vi "AlliGator Update Phasor Plot Image v2.vi"(5 "Image Control Refnum":T1 caption="Phasor Plot Display Refnum", 7 "Phasor Plot Color Scale":refnum<vi>, 8 "Error In":errorcluster, 9 "Phasor Plot Image Elements to Update":string[](array[string]), 10 "AlliGator Internal Variables DVR":refnum<data-value>, 11 "Phasor Plot Display Range Refnum":refnum<vi>) -> (0 "Error Out":errorcluster, 1 "Message":string, 2 "AlliGator Internal Variables DVR":refnum<data-value>)   [LabVIEW 2021, in "AlliGator Phasor Plot.lvlib"]
doc: "Updates the Phasor Plot image including its overlays."
uses:
  AlliGator Phasor Plot.lvlib
  AlliGator Internal Variables v2.ctl
  <vilib>/vision/Image Controls.llb/IMAQ Image.ctl
  AlliGator Gate Image Set.ctl
  AlliGator FLI Dataset Type.ctl
  AlliGator Data Series Type.ctl
  AlliGator Dataset Channel.ctl
  AlliGator Gate Arithmetic.ctl
  AlliGator Displayed Image.ctl
  Image/Named ROI Description.ctl
  AlliGator Decay Metadata v3.ctl
  AlliGator Decay Background Subtraction Info.ctl
  AlliGator Baseline Subtraction Method.ctl
  Graphs/XY Graph/XY Graph Plot Shift Parameters.ctl
  Graphs/XY Graph/XY Graph Plot Shift Method.ctl
  AlliGator Decay Extrapolation Parameters.ctl
  Phasor/Calibration Phasor (m, phi).ctl
  Phasor/Phasor Reference Series.ctl
  Phasor/Phasor Calibration Map v2.ctl
  Phasor/Phasor (g, s).ctl
  AlliGator Raw Phasor Plot Data v4.ctl
  Phasor/Phasor Standard Deviation Options.ctl
  AlliGator Phasor Multi-Harmonic Data.ctl
  Phasor/Phasor Harmonic Data.ctl
  AlliGator Decay Fit Options & Parameters v2.ctl
  Fits/IRF(X)PSED/Decay Fit Options v2.ctl
  Fits/Decay Convolution/Decay Model.ctl
  Fits/Residual Type.ctl
  Fits/IRF(X)PSED/Fit Weights Type.ctl
  Fits/Non-linear Fitting Method v2.ctl
  Fits/Fit Calculation Method.ctl
  Fits/Non-linear Fitting Algorithm.ctl
  AlliGator Decay Fit Parameter Constraints 2.ctl
  Fits/IRF(X)PSED/Decay Fit Parameters In List.ctl
  Fits/IRF(X)PSED/MLE Baseline Offset Type.ctl
  AlliGator Decay Preprocessing Parameters.ctl
  Fits/IRF(X)PSED/Decay Fit Parameters & Derived Quantities List.ctl
  Image/Image Control Refnum.ctl
  AlliGator Variables List.ctl
  a24687bc-c119-402d-9a1a-602e9bf75a15.vi
  Variant/Variant to Data/Variant to U16.vi
  AlliGator Phasor Calibration.lvlib
  AlliGator GUI.lvlib
  AlliGator Settings.lvlib
  Time/Time.lvlib
  AlliGator Globals, Variables & Constants.lvlib
  Variant/Variant to Data/Variant to Data.lvlib
  Phasor/Phasor.lvlib
  7bec4d3f-1ec9-40da-bd4c-cfd082c5c359.vi
  Image/Image.lvlib
  AlliGator Decay Preprocessing.lvlib
  Graphs/XY Graph/XY Graph Add-Ons.lvlib
  AlliGator Phasor Graph.lvlib
  AlliGator Files.lvlib
  AlliGator Internal Variables.lvlib
  AlliGator Source Image.lvlib
  Fits/Fits.lvlib
  AlliGator Decay Fit.lvlib
  AlliGator Decay Fit Parameter Map.lvlib
  AlliGator Dual-Channel Datasets.lvlib
panel:
  out "CPU (s)":dbl
  # "see the AlliGator License on the block diagram (Ctrl+E or Window:Show Block Diagram)"
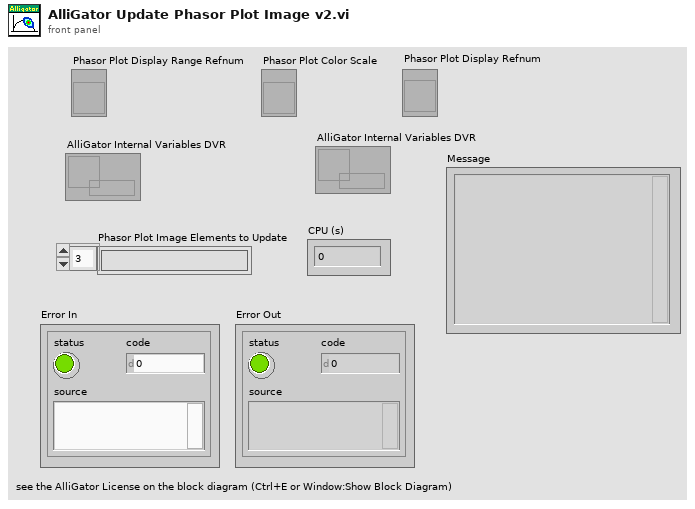
[diagram p1: front panel]
types:
  T1 = typedef "Image.lvlib/Image Control Refnum.ctl" = refnum<vi>
  T2 = typedef "AlliGator Globals, Variables & Constants.lvlib/AlliGator Variables List.ctl" = enum16{"---- GUI ----", "Initialization Status", "State Indicators Refnum", "Original AlliGator Menu Items", "Current Action Loop State", "Script in progress", "Playback", "Loop Playback", "Search ROI Used", "Search ROI", "Decay Graph Max Legend Size", "Intensity Graph Max Legend Size", "Decay Statistics Graph Max Legend Size", "Phasor Graph Max Legend Size", "Phasor Ratio Graph Max Legend Size", "Lifetime Graph Max Legend Size", "---- Files ----", "Export Dataset Frames as Individual Files", "Show Batch Export Help Balloons", "Frames in Dataset", "ptu File Frame Start Indices", "Current Frame in Dataset", "Current Frame Timestamp", "------ Python Plugins ------", "Python Plugins Information", "Python Session", "Valid Python Session?", "---- Source Image ----", "Dataset Loaded", "Dataset Metadata", "Dataset Channel", "Dataset Data Description", "Background Dataset Metadata", "Background Dataset Channel", "Background Dataset Data Description", "Background File Subtraction", "Background File Path", "Background File Pile-up Correction", "Background File Pixel Well Capacity", "Background File Scaling Factor", "Source Image ROIs", "Current Source Image ROI", "Source Image ROI Event Refnum", "X_Source Image Display Range", "X_Source Image Palette Information", "Source Image Palette List", "Source Image Scale", "Current Dataset Load Settings", "Source Image:ROI Overlay Color", "---- Image Profile Window ----", "Image Profile:Overlay ROI in Source Image", "Image Profile Window Event Refnum", "Image Profile:IntensityType", "Image Profile:Intensity Average Type", "Image Profile:Intensity-weighted SDV", "Image Profile:Box Profile Type", "Image Profile Window Open", "Image Profile:Plotted Fit Parameter", "X_Type of Displayed Image", "X_Time Gate Slider", "Dataset Path", "Source Image Overlay to Erase", "Is Displayed Image Accumulated", "White Light Image Modified", "Mask Image Modified", "Macrotime Gate Separation", "------ Phasor Graph -------", "Phasor Graph:Show Line", "---- Phasor Plot ---", "Phasor Plot Parameters Changed", "FLI Dataset Modified since last Phasor Plot Calculation", "Phasor Harmonics Data", "Selected Phasor Harmonics", "Phasor Harmonic Manager Event Refnum", "Phasor Plot ROIs", "Current Phasor Plot ROI", "Phasor Plot ROI Event Refnum", "Phasor Plot Image Reference Points", "Phasor Plot Computed", "Phasor Plot Palette Information", "Phasor Plot Palette List", "Phasor Ratio Palette Information", "Phasor Ratio Palette List", "Phasor Image Scale", "Phasor Plot Image Overlay to Erase", "Phasor Plot Image Elements to Update", "Current Phasor Plot Calculation Parameters", "Current Phasor Calibration Options", "Reset Cumulated Phasor Plot", "Phasor Ratio Reference 1", "Phasor Ratio Lifetime Reference 1", "Phasor Ratio Reference 1 Frequency", "Phasor Ratio Reference 2", "Phasor Ratio Lifetime Reference 2", "Phasor Ratio Reference 2 Frequency", "---- Decay Analysis ----", "Number of Selected Decays to Fit", "LS Fit Results", "LAR Fit Results", "BS Fit Results", "Last Decay Max - Min", "Best Fit Parameters", "Best Fit Parameter Names", "Actual Size X", "Actual Size Y", "Binning X", "Binning Y", "Actual # Gates", "Dataset Number", "Gates to...", "Gates Skipped", "Gates to keep", "Gate Step", "Gate Separation", "Reversed Gates", "Pile-up Correction", "Pixel Well Capacity", "Background Subtracted", "Background Subtraction Method", "Background Definition Range", "Background File (deprecated)", "Number of Dataset Accumulated", "Array of Accumulated Dataset Paths", "Do Averaged Datasets", "Destination File Path", "Process Plot Target", "Use 1/D as Phasor Frequency", "---- Decay Fit Parameter Map -----", "Decay Fit Parameter Map Palette Information", "Decay Fit Parameter Map Palette List", "Local Decay Graph Window Event Refnum", "------- Local Decay Window ---------", "Use normalized IRF for convolution", "----- Miscellaneous ----", "Skippable Dialog Windows Status"}
  T3 = typedef "AlliGator Internal Variables.lvlib/AlliGator Internal Variables v2.ctl" = cluster{"Displayed Image":T4, "White Light Image":T4, "Mask Image":T4, "ROI Mask Image":T4, "Current Dataset Images 1":T5, "Background Dataset Images 1":T5, "Current Dataset Images 2":T5, "Background Dataset Images 2":T5, "Current Dataset Arithmetic Images":T5, "Accumulated Dataset Images 1":T5, "Accumulated Dataset Images 2":T5, "Accumulated Dataset Arithmetic Images":T5, "Phasor Plot Image":T4, "Decay Fit Parameter Map Image":T4, "Single Data Point Path":path, "White Light Image Path":path, "Mask Image Path":path, "Time-Series Folder":path, "[Time-Series Paths]":path[], "Current Dataset":i32, "Single Dataset Type":T6, "Current Folder":string, "AlliGator Data Series Type":T7, "# Datasets":i32, "Dual-Channel Dataset":bool, "Selected Channel Name":string, "Dataset Channel":T8, "Channel Arithmetic":T9, "Dual-Channel Background Dataset":bool, "Background Channel":T8, "Dual-Channel Accumulated Dataset":bool, "Start Time":dbl, "[Time-Series Timestamps]":dbl[], "[Intensity Corrections]":dbl[], "Time Series Script":bool, "Type of Displayed Image":T10, "Gate Image Slide":u16, "# Gates":i32, "ROIs":T11[], "ROI Decay":cluster{"t Array":dbl[], "I Array":dbl[]}, "Valid Decay":bool, "Decay  Metadata":T13, "Reference Decay Plot Name":string, "Reference Decay":cluster{"t Array":dbl[], "I Array":dbl[]}, "Decay Shift Plot":cluster{"Time Stamps":dbl[], "Decay Shifts":dbl[]}, "[Decays Max Values]":sgl[], "[Decays Min Values]":sgl[], "Calibration Phasor":T19, "Calibration Phasor Series":T20, "Phasor Calibration Map":T21, "Calibration Map MD5 Digest":string, "Last Raw Phasor":T22, "Last Calibrated Phasor":T22, "Last Calibrated Phasor SDV":T22, "Phasor Graph:Phasor Plot":cluster{"g Array":dbl[], "s Array":dbl[]}, "Phasor Graph:Phasor SDV Plot":cluster{"g Array":dbl[], "s Array":dbl[]}, "[Phasor Graph:Raw Phasor Plots]":T23[], "Phasor Plot locked to Ref 1":i32, "[Phasor Plot(s) locked to Ref 1]":i32[], "[Phasor Plot(s) locked to Ref 2]":i32[], "[Pixel Phasors]":T22[], "[[Sum Image]]":dbl[][], "[[CSG Phasors]]":csg[][], "[[Valid Pixel?]]":bool[][], "I/m/phi Dataset":cluster{"I/m/phi Dataset?":bool, "Base Frequency":dbl[unit], "Harmonic Orders":u8[]}, "Multi Phasor Plot Data":T25, "Decay Fit Options & Parameters":T27, "Fit Options: Decay Preprocessing Parameters":T38, "Fit Options: Reference Decay":cluster{"t Array":dbl[], "I Array":dbl[]}, "Is Full Image Parameters Map":bool, "Is Single-Pixels Parameters Map":bool, "NLSF Parameters Map X Resolution":i32, "NLSF Parameters Map Y Resolution":i32, "[Single Decay Fit Parameters]":dbl[], "Fit Model":T29, "[[Multiple Decays Fit Parameters]]":dbl[][], "[[Multiple Decays Fit Parameter SDVs]]":dbl[][], "[[IRFs]]":dbl[][], "IRF Array Time Axis":dbl[], "Decay Array Time Axis":dbl[], "[Decay Fit Parameter Names]":T39[], "[[Phasor Ratios]]":dbl[][], "[[Average Lifetimes]]":dbl[][], "Amplitude Weighted Average Lifetime":bool, "[Decay Sum]":dbl[], "[[User-defined Quantities]]":dbl[][], "User-defined Quantity":string}
  T4 = typedef "IMAQ Image.ctl" = refnum<image>
  T5 = typedef "AlliGator Files.lvlib/AlliGator Gate Image Set.ctl" = cluster{"SGL Image Max":T4, "SGL Image Sum":T4, "SGL Gate Images":T4[], "SGL Image Min":T4}
  T6 = typedef "AlliGator Files.lvlib/AlliGator FLI Dataset Type.ctl" = enum16{"HDF5 FLI Dataset", "Gate Image Folder", ".sdt FLI Dataset (Becker & Hickl)", ".ptu FLI Dataset (PicoQuant)", "SS1 FLI Dataset", "SS2 FLI Dataset", "I/m/phi Dataset", ".bin FLI Dataset (PicoQuant Binned)", ".bin FLI Dataset (Piccolo Binned)"}
  T7 = typedef "AlliGator Files.lvlib/AlliGator Data Series Type.ctl" = enum16{"Not a Supported Series", "Gate Images Folder Series", "SwissSPAD 2 Dataset Series", "B&H FLI Dataset Series", "PicoQuant PTU FLI Dataset Series", "PicoQuant BIN FLI Dataset Series", "Piccolo hist BIN FLI Dataset Series", "HDF5 FLI Dataset Series"}
  T8 = typedef "AlliGator Dual-Channel Datasets.lvlib/AlliGator Dataset Channel.ctl" = enum16{"G2", "INT"}
  T9 = typedef "AlliGator Settings.lvlib/AlliGator Gate Arithmetic.ctl" = enum16{"None", "INT-G2", "G2/INT*<INT>", "(1 - G2/INT)*<INT>"}
  T10 = typedef "AlliGator Source Image.lvlib/AlliGator Displayed Image.ctl" = enum16{"Single Gate", "Sum of All Gates", "Max of All Gates", "Min of All Gates", "-", "White Ligth Image", "Mask Image"}
  T11 = typedef "Image.lvlib/Named ROI Description.ctl" = cluster{"ROI Descriptor":T12, "ROI Name":string, "Overlay Color":u32}
  T12 = typedef "ROI Descriptor" = cluster{"Global Rectangle":i32[], "Contours":cluster{"ID":enum32{"External", "Internal"}, "Type":u32, "Coordinates":i32[]}[]}
  T13 = typedef "AlliGator Phasor Graph.lvlib/AlliGator Decay Metadata v3.ctl" = cluster{"ROI Descriptor":T12, "ROI Center":cluster{"X":i32, "Y":i32}, "Decay Background Subtraction Info":T14, "Decay Reverted":bool, "Decay Smoothened":bool, "Decay Straightened":bool, "Fitted Tau (Decay Straightening)":dbl, "Decay Shift Parameters":T16, "Decay Shifted":bool, "Decay Extrapolated":bool, "Decay Extrapolation Parameters":T18, "Decay Normalized":bool, "Fold Decay":bool, "# Folds":u32}
  T14 = typedef "AlliGator Decay Analysis.lvlib/AlliGator Decay Preprocessing.lvlib/AlliGator Decay Background Subtraction Info.ctl" = cluster{"Laser Period":dbl[unit], "Gate Duration":dbl[unit], "Baseline Subtraction Method":T15, "Background Definition Range":cluster{"Min Gate":dbl[unit], "Max Gate":dbl[unit]}, "Total Intensity w/o Bkgd Subtraction":dbl, "Bkgd-subtracted Intensity (exp)":dbl, "# Data Points":i32, "Background/Gate":dbl, "Fitted Lifetime":dbl[unit], "Bkgd-subtracted Intensity (theo)":dbl}
  T15 = typedef "AlliGator Decay Analysis.lvlib/AlliGator Decay Preprocessing.lvlib/AlliGator Baseline Subtraction Method.ctl" = enum16{"Mean", "Min", "Square Gated Single-Exponential", "File", "Constant"}
  T16 = typedef "XY Graph Add-Ons.lvlib/XY Graph Plot Shift Parameters.ctl" = cluster{"Type":T17, "Shift":dbl[unit], "Threshold":dbl, "Rotate":bool}
  T17 = typedef "XY Graph Add-Ons.lvlib/XY Graph Plot Shift Method.ctl" = enum16{"Default", "CFD", "Threshold", "Cross-Correlation"}
  T18 = typedef "AlliGator Decay Analysis.lvlib/AlliGator Decay Preprocessing.lvlib/AlliGator Decay Extrapolation Parameters.ctl" = cluster{"Additional Points":u32, "Head Fraction":dbl, "Fitted Tau":dbl, "Use Periodicity":bool, "Use Cursors":bool, "Tail Fraction":dbl}
  T19 = typedef "Phasor.lvlib/Calibration Phasor (m, phi).ctl" = cluster{"m":dbl, "phi":dbl, "Phasor Frequency":dbl[unit], "Reference Lifetime":dbl[unit]}
  T20 = typedef "Phasor.lvlib/Phasor Reference Series.ctl" = cluster{"m Array":dbl[], "phi Array":dbl[], "Phasor Frequency":dbl[unit], "Calibration Lifetime":dbl[unit]}
  T21 = typedef "Phasor.lvlib/Phasor Calibration Map v2.ctl" = cluster{"Phasor Frequency":dbl[unit], "Calibration Lifetime":dbl[unit], "ROI Centers":cluster{"X":i32, "Y":i32}[], "ROI Descriptors":T12[], "Map Resolution X":i32, "Map Resolution Y":i32, "z Array":cdb[]}
  T22 = typedef "Phasor.lvlib/Phasor (g, s).ctl" = cluster{"g":dbl, "s":dbl}
  T23 = typedef "AlliGator Phasor Graph.lvlib/AlliGator Raw Phasor Plot Data v4.ctl" = cluster{"Phasor Plot Name":string, "Raw Phasor Plot":T22[], "Phasor Frequency":dbl[unit], "[Decay Metadata]":T13[], "Raw Phasor Plot SDV":T22[], "Phasor SDV Options":T24, "[Calibration Phasor]":T19[]}
  T24 = typedef "Phasor.lvlib/Phasor Standard Deviation Options.ctl" = cluster{"Compute Estimated SDV":bool, "# Replicas":u32, "Use Estimated Average Phasor":bool}
  T25 = typedef "AlliGator Phasor Plot.lvlib/AlliGator Phasor Multi-Harmonic Data.ctl" = cluster{"Base Frequency":dbl[unit], "# Harmonics":u8, "Harmonic Orders":u8[], "Phasor Plot Settings Checksum":u64, "Phasor Harmonic Data Array":T26[]}
  T26 = typedef "Phasor.lvlib/Phasor Harmonic Data.ctl" = cluster{"Phasor Harmonic Name":string, "Phasor Plot Settings Checksum":u64, "Phasor Frequency":dbl[unit], "Base Frequency":dbl[unit], "Harmonic Order":u8, "Phasor Plot Parameters":string, "Phasor Array [[CSG]]":csg[][], "Dataset File Path":path}
  T27 = typedef "AlliGator Decay Fit Parameter Map.lvlib/AlliGator Decay Fit Options & Parameters v2.ctl" = cluster{"SYNC Period":dbl[unit], "Fit Options":T28, "Fit Parameter Constraints":T35[], "MLE Baseline Offset":dbl, "MLE Baseline Offset Type":T37}
  T28 = typedef "Fits.lvlib/Decay Fit Options v2.ctl" = cluster{"Show Fit Residuals":bool, "Fit Model":T29, "Residual Type":T30, "Max Decay Percentile":dbl, "Min Decay Percentile":dbl, "Show Full Decay":bool, "Weights":T31, "Fitting Method":T32, "Compute Parameter Uncertainties":bool, "Periodic Boundaries":bool, "Model Calculation":T33, "Period":dbl[unit], "Termination Criteria":cluster{"Max Iterations":i32, "Max Function Calls":i32, "Max Time":dbl[unit], "Function Tolerance":dbl, "Parameter Tolerance":dbl, "Gradient Tolerance":dbl, "Min Lambda":dbl, "Max Lambda":dbl, "Initial Tick Count":u32}, "Offset Resolution":dbl[unit], "Use Local IRF":bool, "Fitting Algorithm":T34}
  T29 = typedef "Fits.lvlib/Decay Model.ctl" = enum16{"1-Exponential", "2-Exponentials"}
  T30 = typedef "Fits.lvlib/Residual Type.ctl" = enum16{"Standard", "Normalized", "Reduced"}
  T31 = typedef "Fits.lvlib/Fit Weights Type.ctl" = enum16{"Unweighted", "1/Variance", "Best of All"}
  T32 = typedef "Fits.lvlib/Non-linear Fitting Method v2.ctl" = enum16{"Least Square", "Least Absolute Residual", "Bisquare", "MLE", "-", "Best of All"}
  T33 = typedef "Fits.lvlib/Fit Calculation Method.ctl" = enum16{"Simulation", "Convolution", "Integration"}
  T34 = typedef "Fits.lvlib/Non-linear Fitting Algorithm.ctl" = enum16{"Levenberg-Marquardt", "Trust-Region Dogleg"}
  T35 = typedef "AlliGator Decay Analysis.lvlib/AlliGator Decay Fit.lvlib/AlliGator Decay Fit Parameter Constraints 2.ctl" = cluster{"Fit Parameter":T36, "Min Value":dbl, "Max Value":dbl, "Global":bool, "Used":bool}
  T36 = typedef "Fits.lvlib/Decay Fit Parameters In List.ctl" = enum16{"Offset", "Baseline", "A_1", "tau_1", "A_2", "tau_2"}
  T37 = typedef "Fits.lvlib/MLE Baseline Offset Type.ctl" = enum32{"Absolute", "Percentage"}
  T38 = typedef "AlliGator Decay Analysis.lvlib/AlliGator Decay Preprocessing.lvlib/AlliGator Decay Preprocessing Parameters.ctl" = cluster{"Background Subtraction":bool, "Straighten Decay":bool, "Reverse Gates":bool, "1-Normalized Decay":bool, "Smoothen Decay":bool, "Smoothing Parameter":dbl, "Shift Decay":bool, "Decay Shift Parameters":T16, "Extrapolate Decay":bool, "Additional Points":u32, "Head Fraction":dbl, "Pixel-Normalize Decay":bool, "Use Periodicity":bool, "Use Cursors":bool, "Tail Fraction":dbl, "Use Decay Pre-Processing":bool, "Fold Decay":bool, "# Folds":u32, "[0-1]-Normalized Decay":bool}
  T39 = typedef "Fits.lvlib/Decay Fit Parameters & Derived Quantities List.ctl" = enum16{"Offset", "Baseline", "A_1", "tau_1", "A_2", "tau_2", "<tau>_a", "f1_a", "f2_a", "<tau>_i", "f1_i", "f2_i", "-", "R^2", "Chi^2"}
  T40 = typedef "AlliGator Phasor Plot.lvlib/AlliGator Phasor Plot Parameters v2.ctl" = cluster{"Phasor Frequency":dbl[unit], "Decay Preprocessing Options & Parameters":T41, "FLI Dataset Modified":bool, "Source Image Settings":cluster{"Low Count Pixels Rejection Options":T43, "High Count Pixels Rejection Options":T44}, "Data Information":cluster{"Gate Width":dbl[unit], "Gate Separation":dbl[unit], "Step (Gate Separation)":i32, "Laser Period":dbl[unit], "SYNC Period":dbl[unit], "Channel Name":u16, "Channel Arithmetic":T9, "Pile-up Correction":bool, "Pixel Well Capacity":u32, "Dataset Scaling Factor":dbl}, "Phasor Plot":cluster{"Phasor Plot Smoothing Options":T45, "Phasor Plot Size":T48, "Selected Image ROI(s)":bool, "All Image ROIs":bool, "Selected Source Image ROI":i32, "Source Image ROIs":T11[]}}
  T41 = typedef "AlliGator Decay Analysis.lvlib/AlliGator Decay Preprocessing.lvlib/AlliGator Decay Preprocessing Options.ctl" = cluster{"Background Subtraction Parameters":T42, "Decay Preprocessing Parameters":T38, "Preprocessing Steps Order":string[]}
  T42 = typedef "AlliGator Decay Analysis.lvlib/AlliGator Decay Preprocessing.lvlib/AlliGator Background Subtraction Parameters.ctl" = cluster{"Background Definition Range":cluster{"Min Gate":dbl[unit], "Max Gate":dbl[unit]}, "Baseline Subtraction Method":T15, "Background Subtraction?":bool, "Background File":path, "Background Constant":dbl, "Background Scaling Factor":dbl, "Background Pile-up Correction":bool, "Background Pixel Well Capacity":u32}
  T43 = typedef "AlliGator Settings.lvlib/AlliGator Low Count Pixels Rejection Options.ctl" = cluster{"Background Low Threshold Factor":dbl, "Fixed Low Background Threshold":dbl, "Reject Low Count Pixels":bool, "Low Percentile":dbl}
  T44 = typedef "AlliGator Settings.lvlib/AlliGator High Count Pixels Rejection Options.ctl" = cluster{"Background High Threshold Factor":dbl, "Fixed High Background Threshold":dbl, "Reject High Count Pixels":bool, "High Percentile":dbl}
  T45 = typedef "AlliGator Phasor Plot.lvlib/AlliGator Phasor Plot Smoothing Options.ctl" = cluster{"Use Phasor Plot Smoothing":bool, "Kernel Type":T46, "Bin":i32, "Algorithm":T47}
  T46 = typedef "Arrays.lvlib/Kernel Type.ctl" = enum16{"Uniform", "Bilinear", "Gaussian"}
  T47 = typedef "Arrays.lvlib/Smoothing Algorithm.ctl" = enum16{"Rapid", "Thorough"}
  T48 = typedef "AlliGator Phasor Plot.lvlib/AlliGator Phasor Plot Size.ctl" = cluster{"H":i32, "V":i32, "Margin":dbl}
  T49 = typedef "Phasor.lvlib/Phasor Calibration Map Characteristics.ctl" = cluster{"Phasor Frequency":dbl[unit], "Calibration Lifetime":dbl[unit], "Map Resolution X":i32, "Map Resolution Y":i32, "Empty Map":bool}
  T50 = typedef "Phasor.lvlib/Phasor Calibration Type.ctl" = enum16{"None", "Single Phasor", "Phasor Series", "Phasor Map"}
  T51 = typedef "AlliGator Phasor Calibration.lvlib/AlliGator Phasor Calibration Options.ctl" = cluster{"Phasor Frequency":dbl[unit], "Phasor Calibration":cluster{"Calibration Lifetime":dbl[unit], "Calibration Type":T50, "Calibration Map Algorithm":T52, "Use Backup Calibration if needed":bool, "Backup Calibration Type":enum16{"Single Calibration", "Nearest Valid Calibration"}}}
  T52 = typedef "AlliGator Phasor Calibration.lvlib/AlliGator Calibration Map Algorithm.ctl" = enum16{"Simple Search", "Min Distance"}
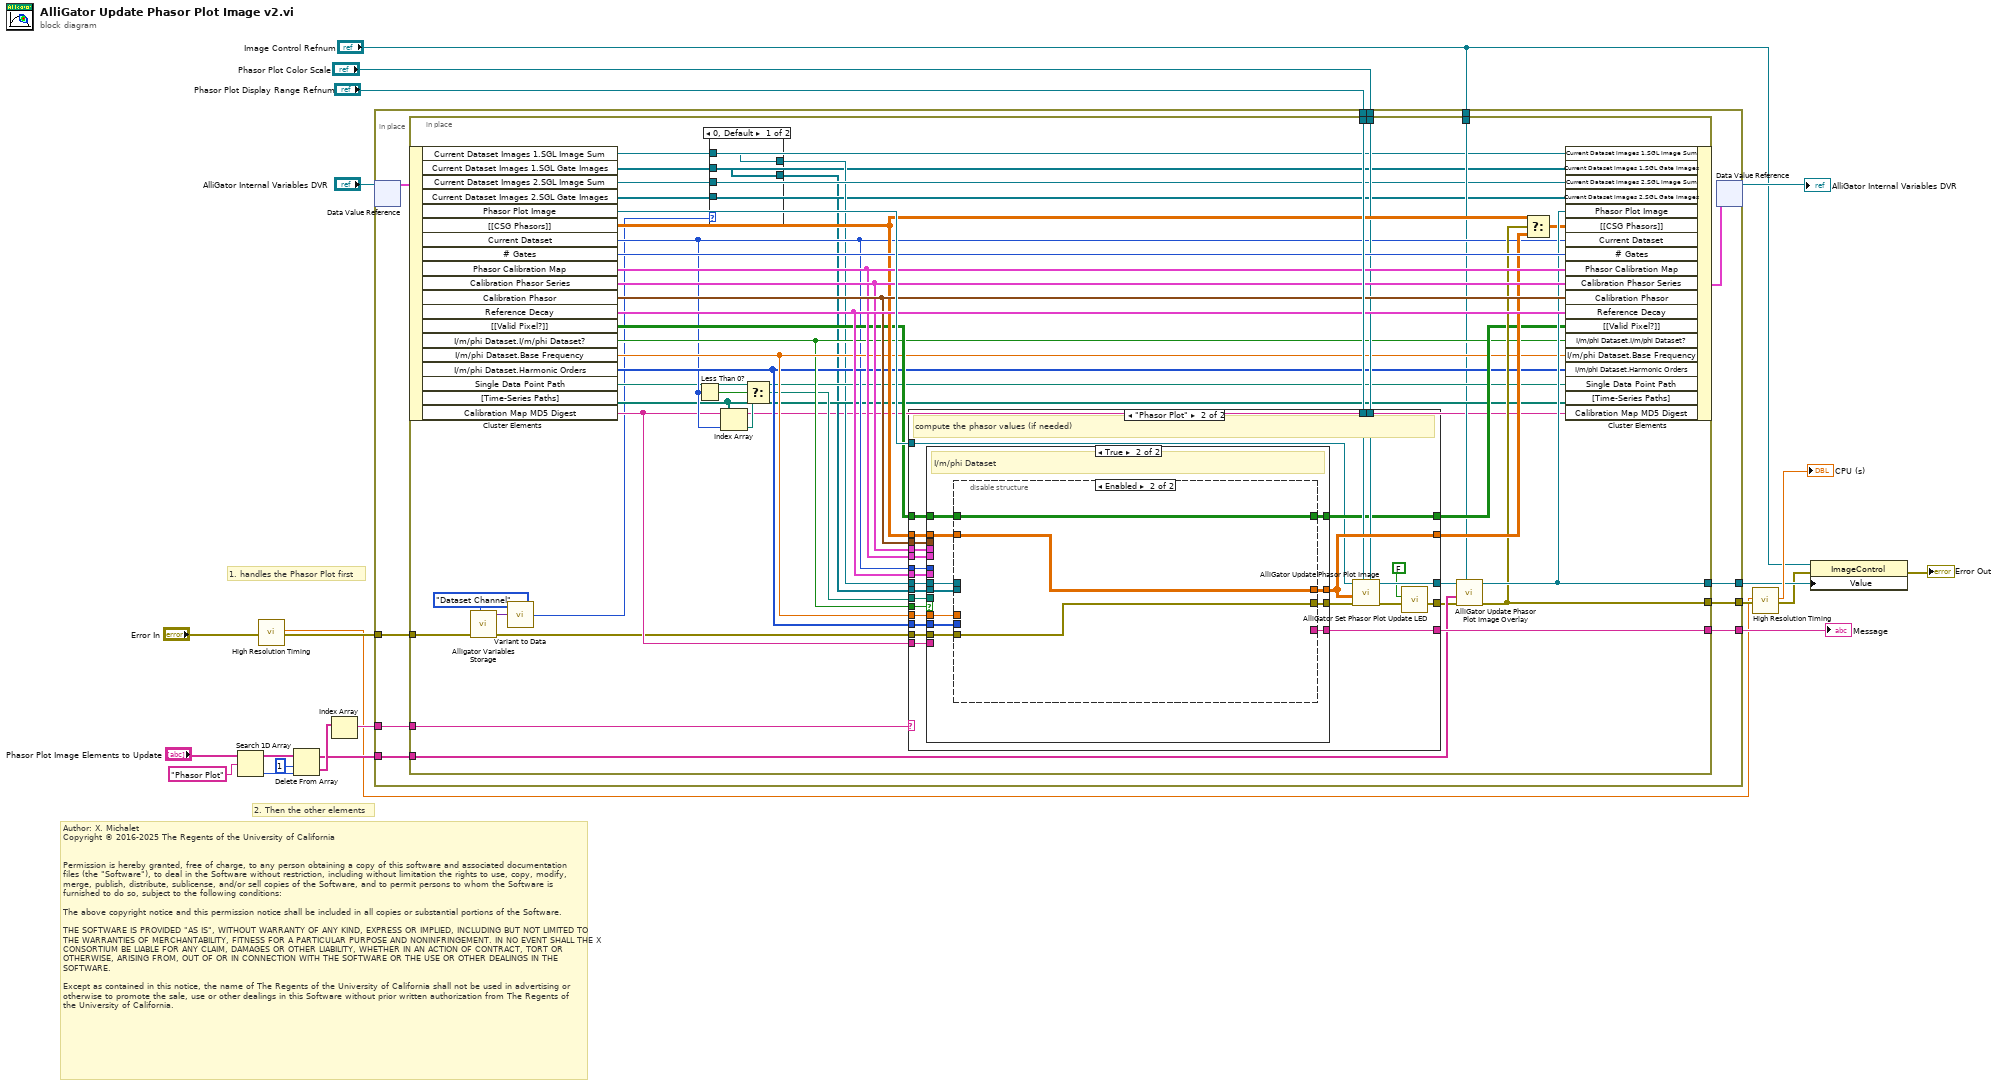
[diagram p0: block diagram]
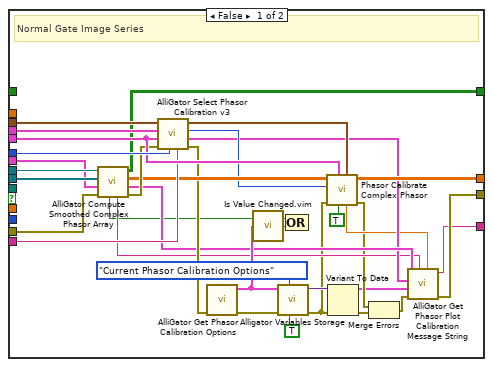
[diagram p4: hidden frame]
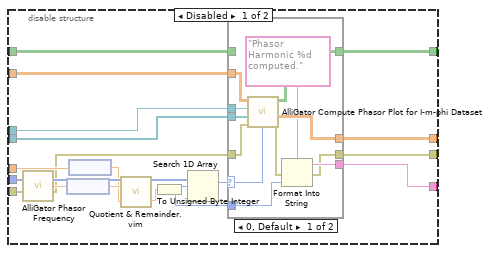
[diagram p5: hidden frame]
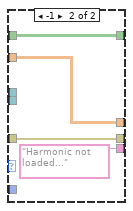
[diagram p6: hidden frame]
diagram:
  # "Author: X. Michalet\nCopyright © 2016-2025 The Regents of the University of California\n \n\nPermission is hereby granted, free of charge, to any person obtaining a copy of this software and associated documentation files (the \"Software\"), to deal in the Software without restriction, including without limitation the rights to use, copy, modify, merge, publish, distribute, sublicense, and/or sell copies of the Software, and to permit persons to whom the Software is furnished to do so, subject to the following conditions:\n\nThe above copyright notice and this permission notice shall be included in all copies or substantial portions of the Software.\n\nTHE SOFTWARE IS PROVIDED \"AS IS\", WITHOUT WARRANTY OF ANY KIND, EXPRESS OR IMPLIED, INCLUDING BUT NOT LIMITED TO THE WARRANTIES OF MERCHANTABILITY, FITNESS FOR A PARTICULAR PURPOSE AND NONINFRINGEMENT. IN NO EVENT SHALL THE X CONSORTIUM BE LIABLE FOR ANY CLAIM, DAMAGES OR OTHER LIABILITY, WHETHER IN AN ACTION OF CONTRACT, TORT OR OTHERWISE, ARISING FROM, OUT OF OR IN CONNECTION WITH THE SOFTWARE OR THE USE OR OTHER DEALINGS IN THE SOFTWARE.\n\nExcept as contained in this notice, the name of The Regents of the University of California shall not be used in advertising or otherwise to promote the sale, use or other dealings in this Software without prior written authorization from The Regents of the University of California."
  # "2. Then the other elements"
  # "1. handles the Phasor Plot first"
  n1 = Search 1D Array(1D array="Phasor Plot Image Elements to Update", element="Phasor Plot") -> (index of element=w19:i32)  [unwired: 1 in]
  n2 = call "High Resolution Timing.vi"("Error In"="Error In") -> ("elapsed (relative) seconds"=w6:dbl, "Error Out"=w7:errorcluster)  [unwired: 16 in, 1 out]
  n3 = Delete From Array(array="Phasor Plot Image Elements to Update", length=1, index=w19) -> (deleted portion=w17:string[], array with subset deleted=w14:string[])
  n4 = Index Array(array=w17) -> (element=w16:string)  [unwired: 1 in]
  n5 = in-place {
    in-place-border: [w32] -> w21
    in-place-border: w16 -> [w31]
    in-place-border: w7 -> [w30]
    in-place-border: [w29] -> w4
    in-place-border: [w28] -> w15
    in-place-border: w14 -> [w27]
    in-place-border: "Phasor Plot Display Range Refnum" -> [w24]
    in-place-border: "Phasor Plot Color Scale" -> [w23]
    in-place-border: "Image Control Refnum" -> [w22]
    n6 = in-place-dvr #1("AlliGator Internal Variables DVR") -> (w26:T3)  [unwired: 1 out]
    n7 = in-place {
      in-place-border: [w74] -> w32
      in-place-border: w31 -> [w73]
      in-place-border: w30 -> [w35]
      in-place-border: [w64] -> w29
      in-place-border: [w60] -> w28
      in-place-border: w27 -> [w72]
      in-place-border: w24 -> [w70]
      in-place-border: w23 -> [w59]
      in-place-border: w22 -> [w45]
      n8 = in-place-cluster #2(w26) -> ("Current Dataset Images 1.SGL Image Sum"=w44:T4, "Current Dataset Images 1.SGL Gate Images"=w41:T4[], "Current Dataset Images 2.SGL Image Sum"=w43:T4, "Current Dataset Images 2.SGL Gate Images"=w40:T4[], "Phasor Plot Image"=w71:T4, "[[CSG Phasors]]"=w61:csg[][], "Current Dataset"=w50:i32, "# Gates"=w65:i32, "Phasor Calibration Map"=w66:T21, "Calibration Phasor Series"=w67:T20, "Calibration Phasor"=w68:T19, "Reference Decay"=w69:cluster{"t Array":dbl[], "I Array":dbl[]}, "[[Valid Pixel?]]"=w58:bool[][], "I/m/phi Dataset.I/m/phi Dataset?"=w53:bool, "I/m/phi Dataset.Base Frequency"=w54:dbl[unit], "I/m/phi Dataset.Harmonic Orders"=w52:u8[], "Single Data Point Path"=w47:path, "[Time-Series Paths]"=w46:path[], "Calibration Map MD5 Digest"=w38:string)
      n9 = call "Alligator Variables Storage.vi"("AlliGator Variable"=AlliGator_Variables_List."Dataset Channel" ("Alligator Variable"), "Error In"=w35) -> ("Error Out"=w34:errorcluster, "Data out"=w36:variant)  [unwired: 7 in, 1 out]
      n10 = call-poly "Variant to Data.vi"("Variant"=w36) -> ("U16 Value"=w33:u16)  [unwired: 8 in]
      n11 = Less Than 0?(x=w50) -> (x < 0?=w51:bool)
      n12 = case shown="0, Default" w33 {
        tunnel: [w76 w78] -> w42
        tunnel: w43 -> [_ w78]
        tunnel: [w75 w77] -> w39
        tunnel: w40 -> [_ w77]
        tunnel: w44 -> [w76 _]
        tunnel: w41 -> [w75 _]
        frame 0, Default {
        }
        frame 1 {
        }
      }
      n13 = Index Array(array=w46, index=w50) -> (element=w49:path)
      n14 = Select(t=w47, s=w51, f=w49) -> (s? t:f=w48:path)
      n15 = case shown="\"Phasor Plot\"" w73 {
        tunnel: w42 -> [_ w108]
        tunnel: [w80 w103] -> w63
        tunnel: w39 -> [_ w107]
        tunnel: [_ w104] -> w74
        tunnel: [w81 w93] -> w55
        tunnel: w71 -> [w82 w84]
        tunnel: [w82 w106] -> w56
        tunnel: w34 -> [w81 w99]
        tunnel: w61 -> [w80 w86]
        tunnel: w70 -> [_ w102]
        tunnel: w68 -> [_ w101]
        tunnel: w67 -> [_ w100]
        tunnel: w66 -> [_ w97]
        tunnel: w50 -> [_ w98]
        tunnel: w69 -> [_ w96]
        tunnel: w59 -> [_ w92]
        tunnel: [w79 w91] -> w57
        tunnel: w58 -> [w79 w87]
        tunnel: w53 -> [_ w90]
        tunnel: w54 -> [_ w89]
        tunnel: w52 -> [_ w88]
        tunnel: w48 -> [_ w85]
        tunnel: w38 -> [_ w83]
        frame "", Default {
          # "keep the current phasor values"
        }
        frame "Phasor Plot" {
          # "compute the phasor values (if needed)"
          n16 = case shown="True" w90 {
            tunnel: w108 -> [w143 w144]
            tunnel: w107 -> [w142 w147]
            tunnel: [w141 w148] -> w105
            tunnel: [w140 w150] -> w104
            tunnel: [w139 w151] -> w103
            tunnel: w101 -> [w138 _]
            tunnel: w100 -> [w137 _]
            tunnel: w99 -> [w136 w149]
            tunnel: w98 -> [w135 _]
            tunnel: w97 -> [w134 _]
            tunnel: w96 -> [w133 _]
            tunnel: [w132 w145] -> w91
            tunnel: w89 -> [_ w153]
            tunnel: w88 -> [_ w154]
            tunnel: w87 -> [_ w146]
            tunnel: w86 -> [_ w152]
            tunnel: w85 -> [_ _]
            tunnel: w83 -> [w131 _]
            frame False {
              # "Normal Gate Image Series"
              n17 = call "AlliGator Compute Smoothed Complex Phasor Array.vi"("error in (no error)"=w136, "Time-Gated Reference Decay"=w133, "Image Array"=w142, "Sum Image"=w143) -> ("error out"=w130:errorcluster, "Phasor Plot Parameters"=w121:T40, "Corrected Complex Phasor Array out (VxH)"=w129:csg[][], "Valid Pixel?"=w132:bool[][], "Message"=w119:string, "Phasor Array updated"=w115:bool)  [unwired: 2 in]
              n18 = call "AlliGator Select Phasor Calibration v3.vi"("Calibration Map MD5 Digest"=w131, "Current Data Set (-1: single)"=w135, "Error In"=w130, "Phasor Calibration Map"=w134, "Calibration Phasor Series"=w137, "Calibration Phasor"=w138) -> ("Error Out"=w126:errorcluster, "Phasor Calibration Map Characteristics"=w120:T49, "Calibration Type Used"=w127:T50, "Calibration Phasor"=w128:T19)  [unwired: 2 in]
              n19 = call "AlliGator Get Phasor Calibration Options.vi"("Error In"=w126) -> ("Error Out"=w117:errorcluster, "Phasor Calibration Options"=w122:T51)  [unwired: 8 in, 1 out]
              n20 = call "Is Value Changed.vim"("value"=w122) -> ("changed or first call?"=w125:bool)
              n21 = call "Alligator Variables Storage.vi"("Get(F)/Set"=TRUE, "AlliGator Variable"=AlliGator_Variables_List."Current Phasor Calibration Options" ("Alligator Variable"), "Error In"=w117, "Data in"=w122) -> ("Error Out"=w112:errorcluster, "Data out"=w114:variant)  [unwired: 5 in, 1 out]
              n22 = Compound Arithmetic op=OR(w115, w125) -> ()  [unwired: 1 out]
              n23 = call "Phasor Calibrate Complex Phasor.vi"("Calibration Phasor"=w128, "Force Calibration (T)"=TRUE, "Phasor Calibration Map"=w134, "Error In"=w112, "Calibration Type Used"=w127, "Complex Phasor Array (VxH)"=w129) -> ("Error Out"=w116:errorcluster, "Corrected Complex Phasor Array (VxH)"=w139:csg[][], "CPU (s)"=w118:dbl)  [unwired: 3 in]
              n24 = Variant To Data(error in=w112, Variant=w114) -> (data=w113:T51, error out=w110:errorcluster)  [unwired: 1 in]
              n25 = Merge Errors(w116, w110) -> (w111:errorcluster)
              n26 = call "AlliGator Get Phasor Plot Calibration Message String.vi"("Calibration CPU (s)"=w118, "Message in"=w119, "error in (no error)"=w111, "AlliGator Phasor Calibration Options"=w113, "Phasor Calibration Map Characteristics"=w120, "Phasor Plot Parameters"=w121) -> ("error out"=w141:errorcluster, "Message out"=w140:string)  [unwired: 4 in]
            }
            frame True {
              # "I/m/phi Dataset"
              n27 = disable-structure shown="Enabled" {
                disable-tunnel: w154 -> [w168 _]
                disable-tunnel: w153 -> [w167 _]
                disable-tunnel: w152 -> [w165 w189]
                disable-tunnel: [w164 w189] -> w151
                disable-tunnel: [w163 _] -> w150
                disable-tunnel: w149 -> [w162 w188]
                disable-tunnel: [w161 w188] -> w148
                disable-tunnel: w147 -> [w160 _]
                disable-tunnel: w146 -> [w158 w190]
                disable-tunnel: [w157 w190] -> w145
                disable-tunnel: w144 -> [w156 _]
                frame Disabled {
                  n28 = call "AlliGator Phasor Frequency.vi"() -> ("Phasor Frequency"=w171:dbl[unit])
                  n29 = node(w171) -> (w170:dbl)
                  n30 = node(w167) -> (w155:dbl)
                  n31 = call "Quotient & Remainder.vim"("y"=w155, "x"=w170) -> ("E(x/y)"=w169:dbl)  [unwired: 1 out]
                  n32 = To Unsigned Byte Integer(number=w169) -> (unsigned 8bit integer=w159:u8)
                  n33 = Search 1D Array(1D array=w168, element=w159) -> (index of element=w166:i32)  [unwired: 1 in]
                  n34 = case shown="0, Default" w166 {
                    selector: w166 -> [w180 _]
                    tunnel: w165 -> [w181 w187]
                    tunnel: [w175 w187] -> w164
                    tunnel: [w179 "Harmonic not loaded..." ("Message")] -> w163
                    tunnel: w162 -> [w183 w185]
                    tunnel: [w177 w185] -> w161
                    tunnel: w160 -> [w182 _]
                    tunnel: w159 -> [w176 _]
                    tunnel: w158 -> [_ w184]
                    tunnel: [w174 w184] -> w157
                    tunnel: w156 -> [w173 _]
                    frame 0, Default {
                      n35 = call "AlliGator Compute Phasor Plot for I-m-phi Dataset.vi"("Harmonic index"=w180, "error in (no error)"=w183, "Image Array"=w182, "Sum Image"=w173, "[[CSG]] Phasor Array in"=w181) -> ("error out"=w178:errorcluster, "[[CSG]] Phasor Array out"=w175:csg[][], "Valid Pixel?"=w174:bool[][])  [unwired: 4 in]
                      n36 = Format Into String(format string="Phasor Harmonic %d computed.", error in=w178, w176) -> (resulting string=w179:string, error out=w177:errorcluster)  [unwired: 1 in]
                    }
                    frame -1 {
                    }
                  }
                }
                frame Enabled {
                }
              }
            }
          }
          n37 = call "AlliGator Update Phasor Plot Image.vi"("Phasor Plot Color Scale"=w92, "Phasor Plot Display Range Refnum"=w102, "error in (no error)"=w105, "Corrected Complex Phasor Array"=w103, "Phasor Plot Image in"=w84) -> ("error out"=w94:errorcluster, "Phasor Plot Image out"=w106:T4)  [unwired: 4 in, 1 out]
          n38 = call "AlliGator Set Phasor Plot Update LED.vi"("error in (no error)"=w94, "Off/On"=FALSE) -> ("error out"=w93:errorcluster)  [unwired: 9 in]
        }
      }
      n39 = call "AlliGator Update Phasor Plot Image Overlay.vi"("Image Control Refnum"=w45, "error in (no error)"=w55, "Overlay List"=w72, "Phasor Plot Image in"=w56) -> ("error out"=w60:errorcluster, "Phasor Plot Image out"=w64:T4)  [unwired: 6 in]
      n40 = Select(t=w61, s=w60, f=w63) -> (s? t:f=w62:csg[][])
      n41 = in-place-cluster #2("Current Dataset Images 1.SGL Image Sum"=w44, "Current Dataset Images 1.SGL Gate Images"=w41, "Current Dataset Images 2.SGL Image Sum"=w43, "Current Dataset Images 2.SGL Gate Images"=w40, "Phasor Plot Image"=w64, "[[CSG Phasors]]"=w62, "Current Dataset"=w50, "# Gates"=w65, "Phasor Calibration Map"=w66, "Calibration Phasor Series"=w67, "Calibration Phasor"=w68, "Reference Decay"=w69, "[[Valid Pixel?]]"=w57, "I/m/phi Dataset.I/m/phi Dataset?"=w53, "I/m/phi Dataset.Base Frequency"=w54, "I/m/phi Dataset.Harmonic Orders"=w52, "Single Data Point Path"=w47, "[Time-Series Paths]"=w46, "Calibration Map MD5 Digest"=w38) -> (w25:T3)
    }
    n42 = in-place-dvr #1(w25) -> (→"AlliGator Internal Variables DVR":refnum<data-value>)  [unwired: 1 out]
  }
  "Message" <- w21
  n43 = call "High Resolution Timing.vi"("relative seconds (NaN)"=w6, "Error In"=w15) -> ("elapsed (relative) seconds"=→"CPU (s)":dbl, "Error Out"=w3:errorcluster)  [unwired: 15 in, 1 out]
  n44 = property class="ImageControl"(reference="Image Control Refnum", error in=w3, "Value"=w4) -> (error out=→"Error Out":errorcluster)  [unwired: 1 out]
